vi "test_shuffle_array.vi"() -> ()   [LabVIEW 2021]
uses:
  acda8cda-a148-3fe5-70ba-265bad15db3f.vi
  73ac5080-7ff9-3fc1-b2ca-39523593ed3f.vi
  929d9f70-b382-3fdc-4057-ce21f6d5de3f.vi
  acda8cda-a148-3fe5-70ba-265bad15db3f.vi/583681f2-f74d-3fed-28b4-9e1d217ae73f.vi
panel:
  out "shuffled string":string
  out "shuffled cards":cluster{"Ring 3":u16, "Ring 4":u16}[](array[cluster])=[{"Ring 3"=0, "Ring 4"=1}, {"Ring 3"=0, "Ring 4"=2}, {"Ring 3"=0, "Ring 4"=3}, {"Ring 3"=0, "Ring 4"=4}, {"Ring 3"=1, "Ring 4"=5}, {"Ring 3"=1, "Ring 4"=6}, {"Ring 3"=1, "Ring 4"=7}, {"Ring 3"=1, "Ring 4"=8}] {"Ring 3" items=["Spade", "Heart", "Club", "Diamond"]; "Ring 4" items=["A"=1, "2"=2, "3"=3, "4"=4, "5"=5, "6"=6, "7"=7, "8"=8, "9"=9, "10"=10, "J"=11, "Q"=12, "K"=13]}
  out "shuffled  strings":string[](array[string])
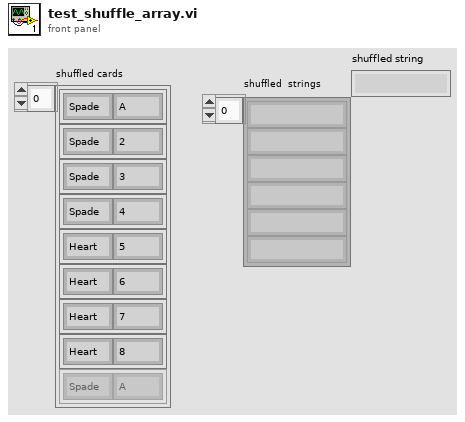
[diagram p1: front panel]
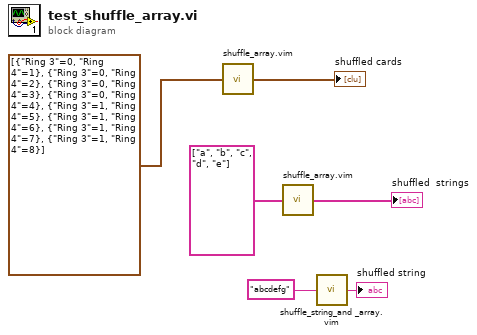
[diagram p0: block diagram]
diagram:
  n1 = call "shuffle_array.vim"("array"=cluster{"Ring 3":u16, "Ring 4":u16}[] [{"Ring 3"=0, "Ring 4"=1}, {"Ring 3"=0, "Ring 4"=2}, {"Ring 3"=0, "Ring 4"=3}, {"Ring 3"=0, "Ring 4"=4}, {"Ring 3"=1, "Ring 4"=5}, {"Ring 3"=1, "Ring 4"=6}, {"Ring 3"=1, "Ring 4"=7}, {"Ring 3"=1, "Ring 4"=8}]) -> ("shuffled array"=→"shuffled cards":cluster{"Ring 3":u16, "Ring 4":u16}[])
  n2 = call "shuffle_array.vim"("array"=string[] ["a", "b", "c", "d", "e"]) -> ("shuffled array"=→"shuffled  strings":string[])
  n3 = call "shuffle_string_and _array.vim"("array"="abcdefg") -> ("shuffled array"=→"shuffled string":string)
